vi "AlGaInPAs_v22b.vi"(2 "Debug Mode":bool, 3 "Elapsed Time(s)":dbl, 4 "State":enum16{"Edit", "Start", "Run", "End", "Idle"}(ring), 5 "Argument List In":string[](array[string])) -> (0 "Status Out":string, 1 "Argument List Out":string[](array[string]))   [LabVIEW 2011]
uses:
  high_level_proc/source_dilution.ctl
  high_level_proc/source_noDilution.ctl
panel:
  in  "Ring":u16(ring)
  out "source array":refnum<vi>[](array[refnum])
  in  "Zn bubbler":T1={"Dilution"=FALSE, "Calculated"=0, "MFC1 flow"=0.0, "MFC2 flow"=10.0, "MFC3 flow"=100.0, "Main"={"Flow"=0.0, "Prep"=FALSE, "Run"=FALSE, "Active"=FALSE, "Name"="Zn"}} caption="Al" {"Main"."Flow" format="%.2f"; "MFC1 flow" format="%.4f"; "MFC3 flow" format="%.1f"; "MFC2 flow" format="%.2f"; "Calculated" items=["Flow", "MFC1", "MFC2", "MFC3"]}
  in  "Al bubbler":T2={"Flow"=0.0, "Prep"=FALSE, "Run"=FALSE, "Active"=FALSE, "Name"="Al"} caption="Al" {"Flow" format="%.2f"}
  in  "Se bubbler":T1={"Dilution"=FALSE, "Calculated"=0, "MFC1 flow"=0.0, "MFC2 flow"=10.0, "MFC3 flow"=100.0, "Main"={"Flow"=0.0, "Prep"=FALSE, "Run"=FALSE, "Active"=FALSE, "Name"="Se"}} caption="Al" {"Main"."Flow" format="%.2f"; "MFC1 flow" format="%.4f"; "MFC3 flow" format="%.1f"; "MFC2 flow" format="%.2f"; "Calculated" items=["Flow", "MFC1", "MFC2", "MFC3"]}
  in  "P bubbler":T2={"Flow"=0.0, "Prep"=FALSE, "Run"=FALSE, "Active"=FALSE, "Name"="P liq"} caption="Al" {"Flow" format="%.2f"}
  in  "As gas":T2={"Flow"=0.0, "Prep"=FALSE, "Run"=FALSE, "Active"=FALSE, "Name"="As gas"} caption="Al" {"Flow" format="%.2f"}
  in  "P gas":T2={"Flow"=0.0, "Prep"=FALSE, "Run"=FALSE, "Active"=FALSE, "Name"="P gas"} caption="Al" {"Flow" format="%.2f"}
  in  "In bubbler":T2={"Flow"=0.0, "Prep"=FALSE, "Run"=FALSE, "Active"=FALSE, "Name"="In"} caption="Al" {"Flow" format="%.2f"}
  in  "Ga bubbler":T1={"Dilution"=FALSE, "Calculated"=0, "MFC1 flow"=0.0, "MFC2 flow"=10.0, "MFC3 flow"=100.0, "Main"={"Flow"=0.0, "Prep"=FALSE, "Run"=FALSE, "Active"=FALSE, "Name"="Ga"}} caption="Al" {"Main"."Flow" format="%.2f"; "MFC1 flow" format="%.4f"; "MFC3 flow" format="%.1f"; "MFC2 flow" format="%.2f"; "Calculated" items=["Flow", "MFC1", "MFC2", "MFC3"]}
  out "prep_done":bool
  out "run started":bool
  out "first":bool=TRUE
  out "is OK?":bool
  in  "prep_time":dbl
  in  "Cancel":bool
  in  "OK":bool
  # "s"
  # "Add pre-run time to run time in editor."
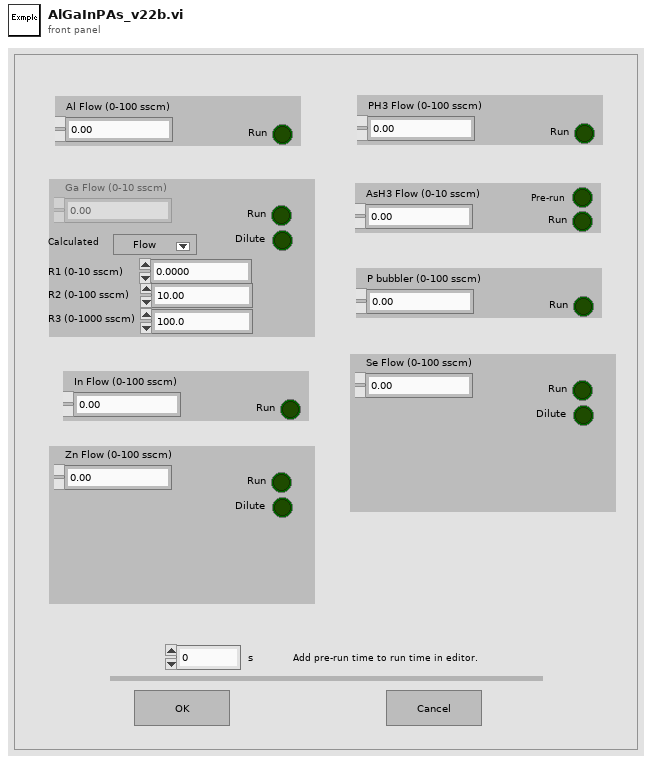
[diagram p1: front panel]
types:
  T1 = typedef "source_dilution.ctl" = cluster{"Dilution":bool, "Calculated":u16, "MFC1 flow":dbl, "MFC2 flow":dbl, "MFC3 flow":dbl, "Main":T2}
  T2 = typedef "source_noDilution.ctl" = cluster{"Flow":dbl, "Prep":bool, "Run":bool, "Active":bool, "Name":string}
  T3 = enum32{"Invalid", "Default", "Floating", "Floating/Auto-Hide", "Modal"}
  T4 = enum16{"Discrete", "Continuous", "Instantaneous", "Finite"}
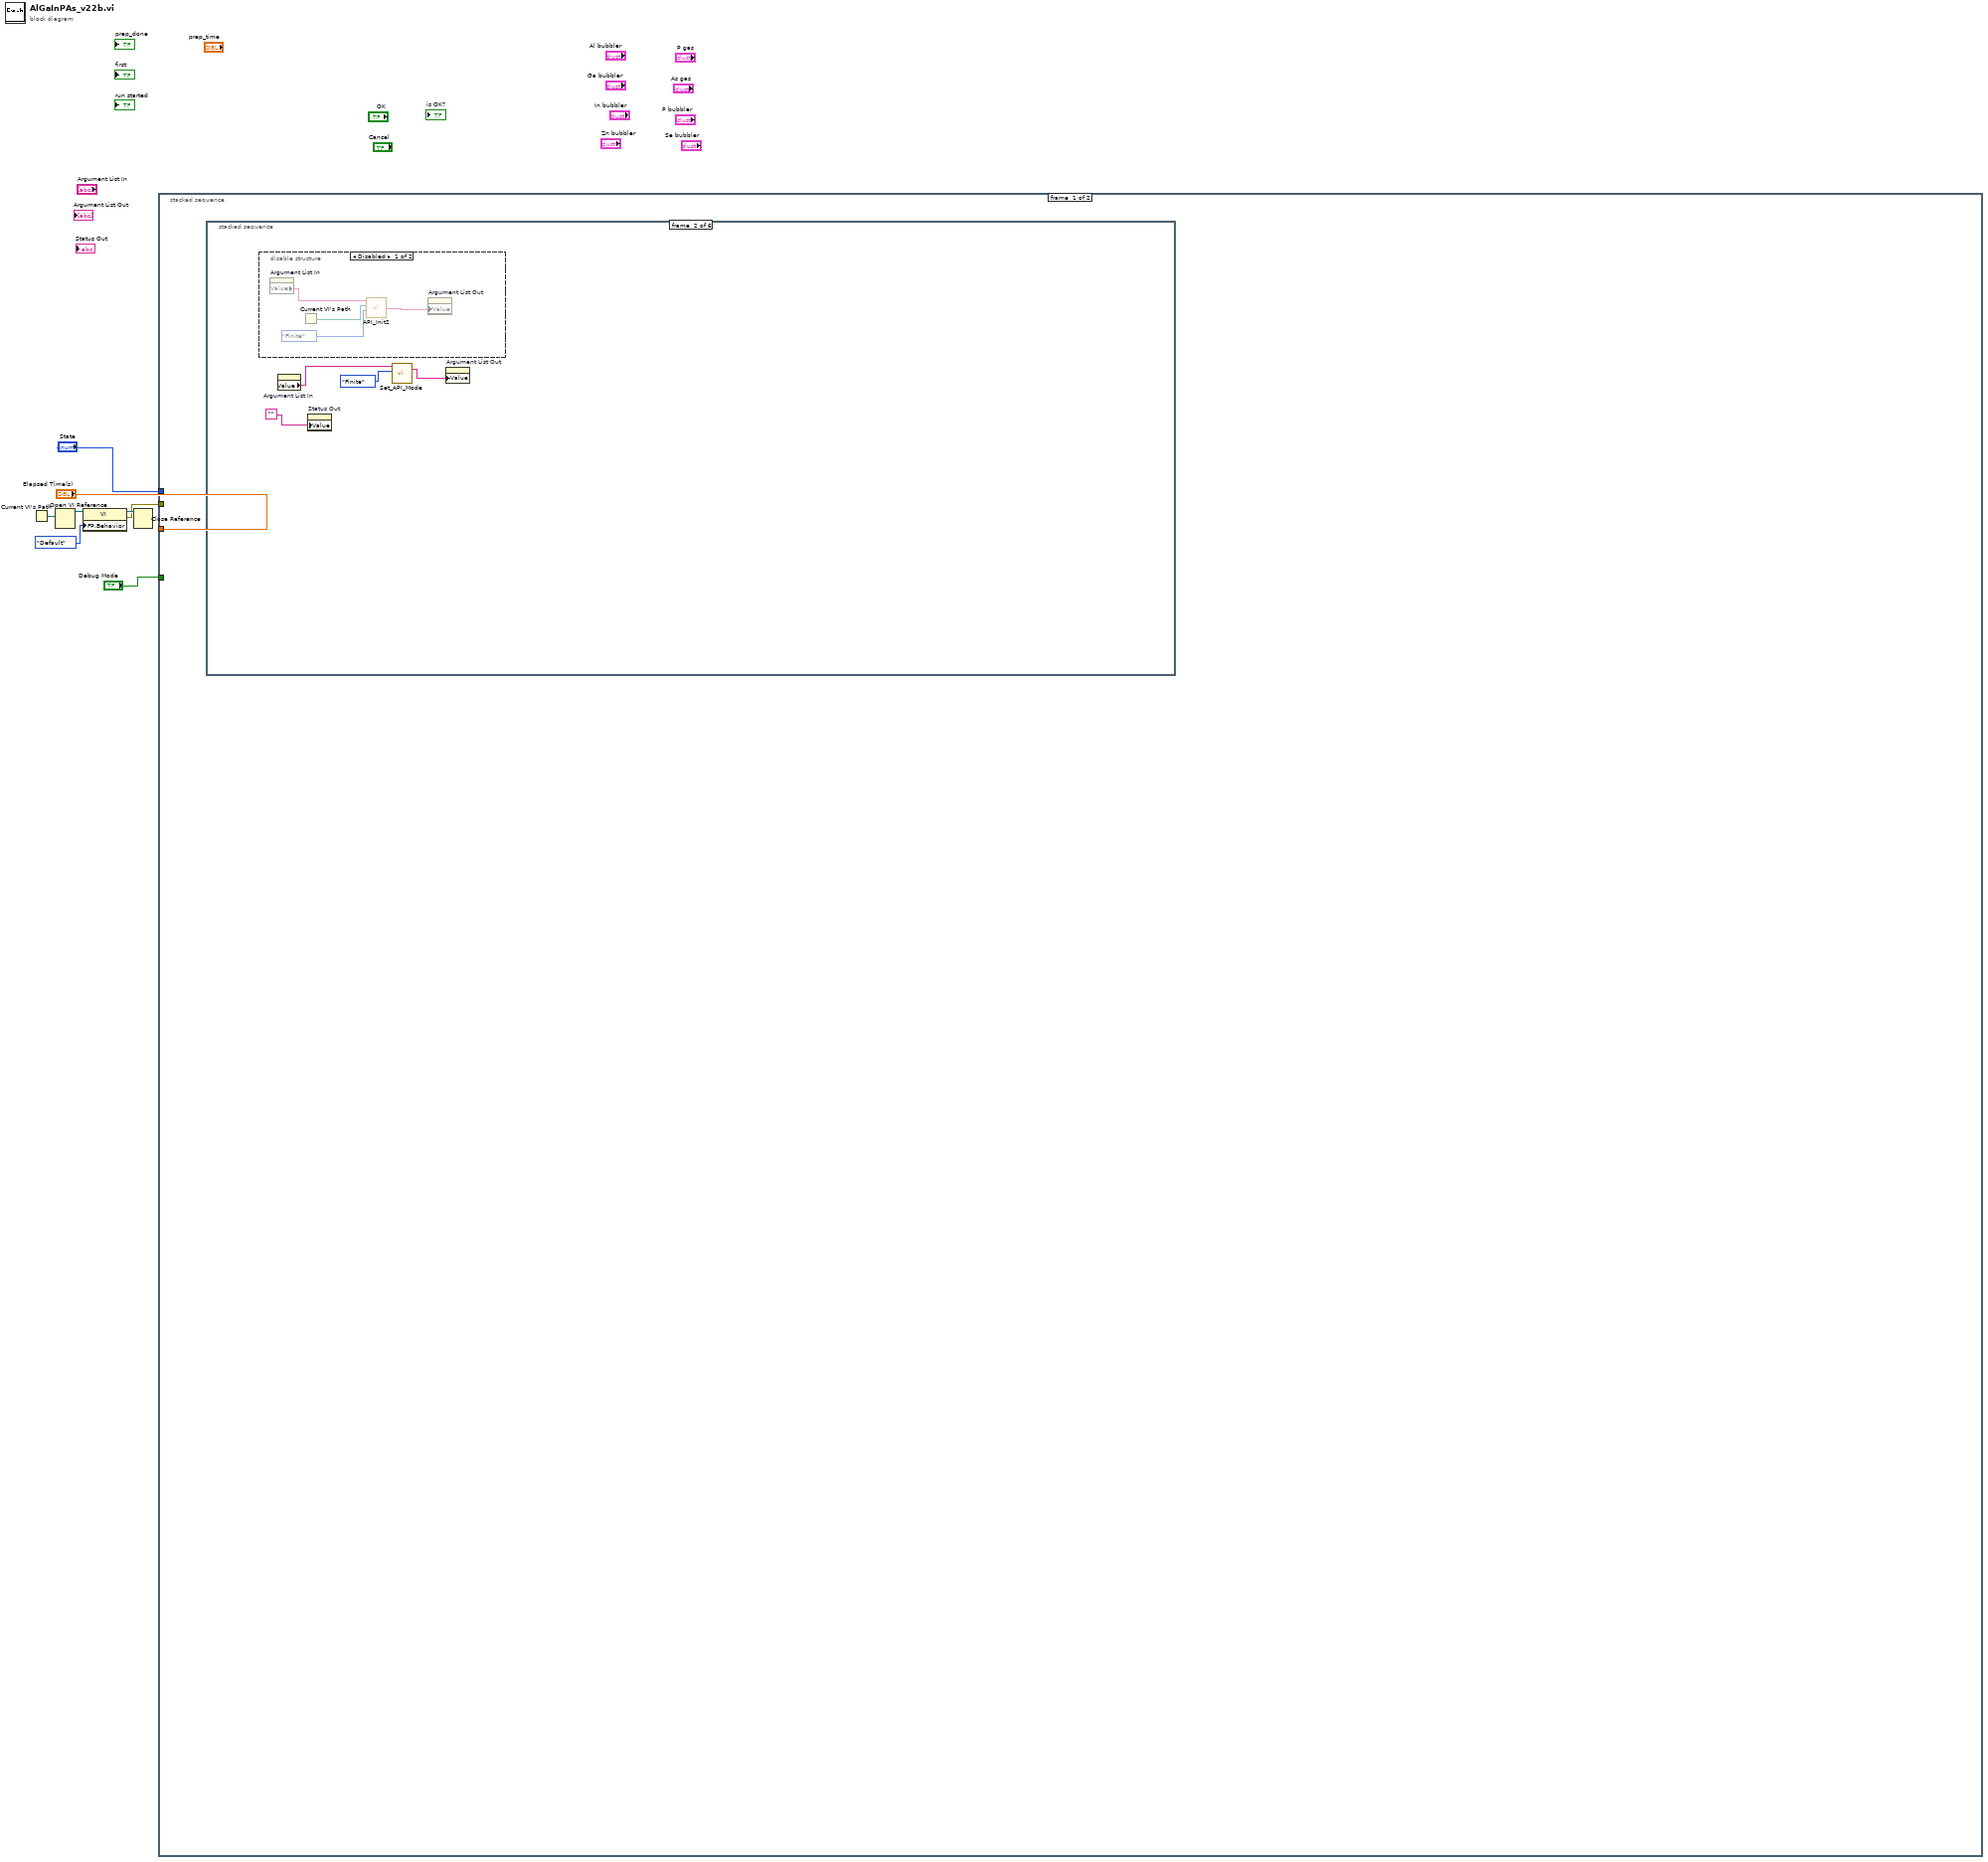
[diagram p0: block diagram]
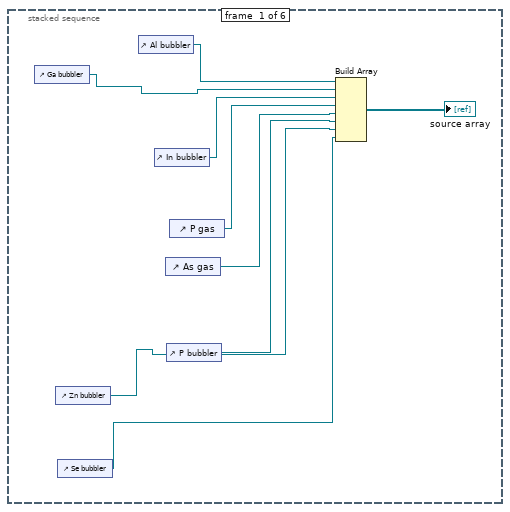
[diagram p2: hidden frame]
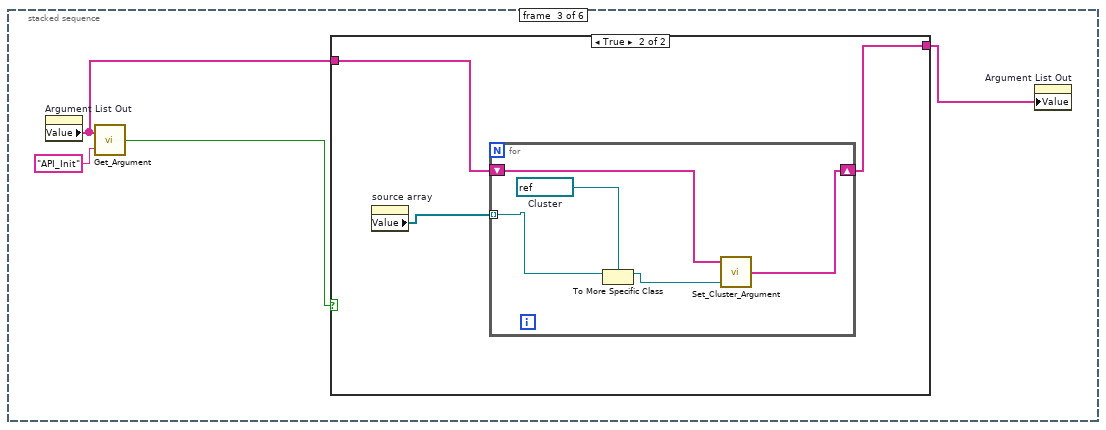
[diagram p4: hidden frame]
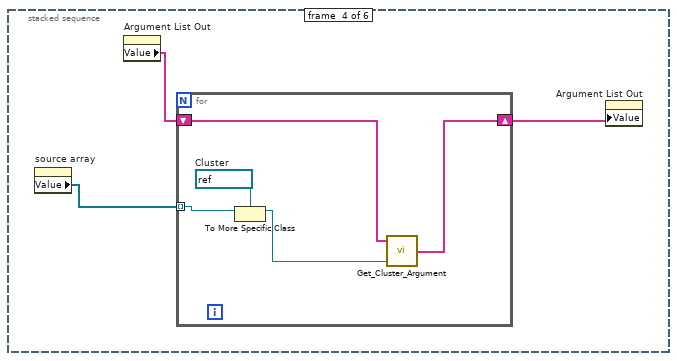
[diagram p6: hidden frame]
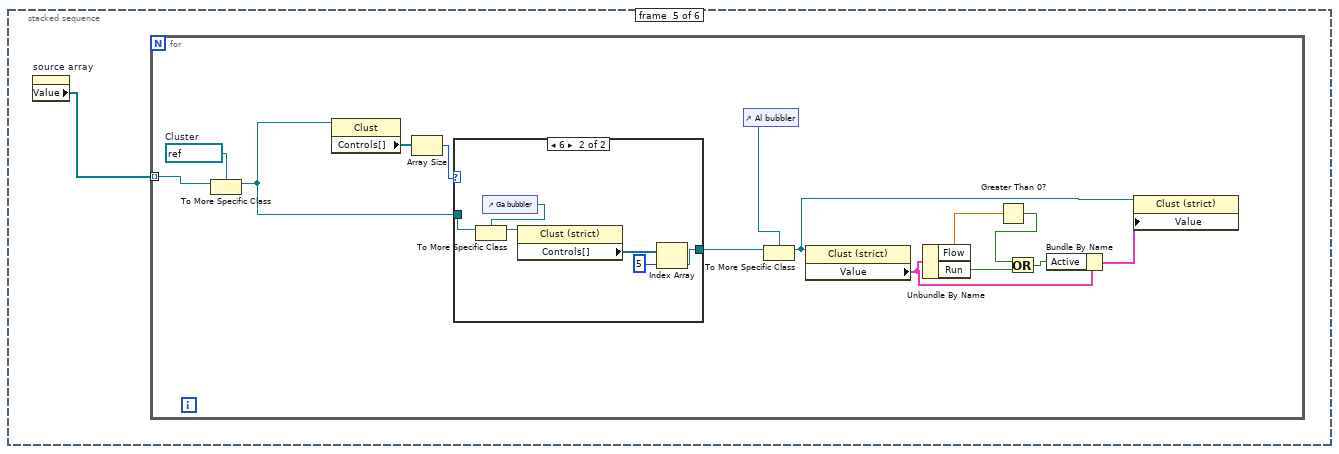
[diagram p7: hidden frame]
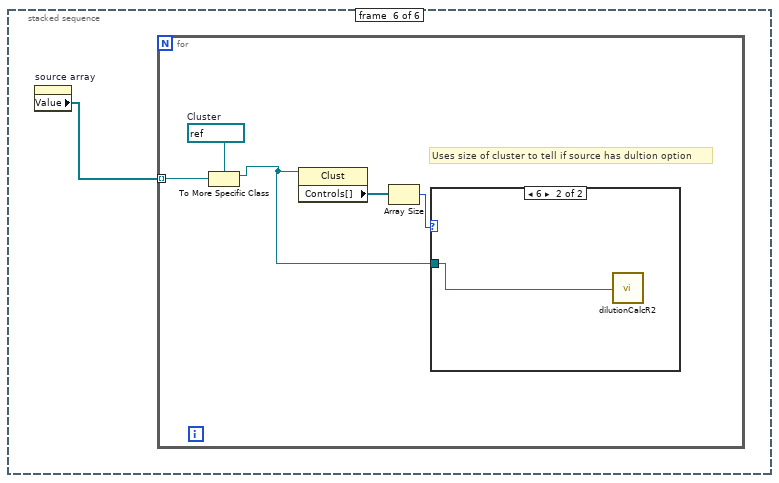
[diagram p9: hidden frame]
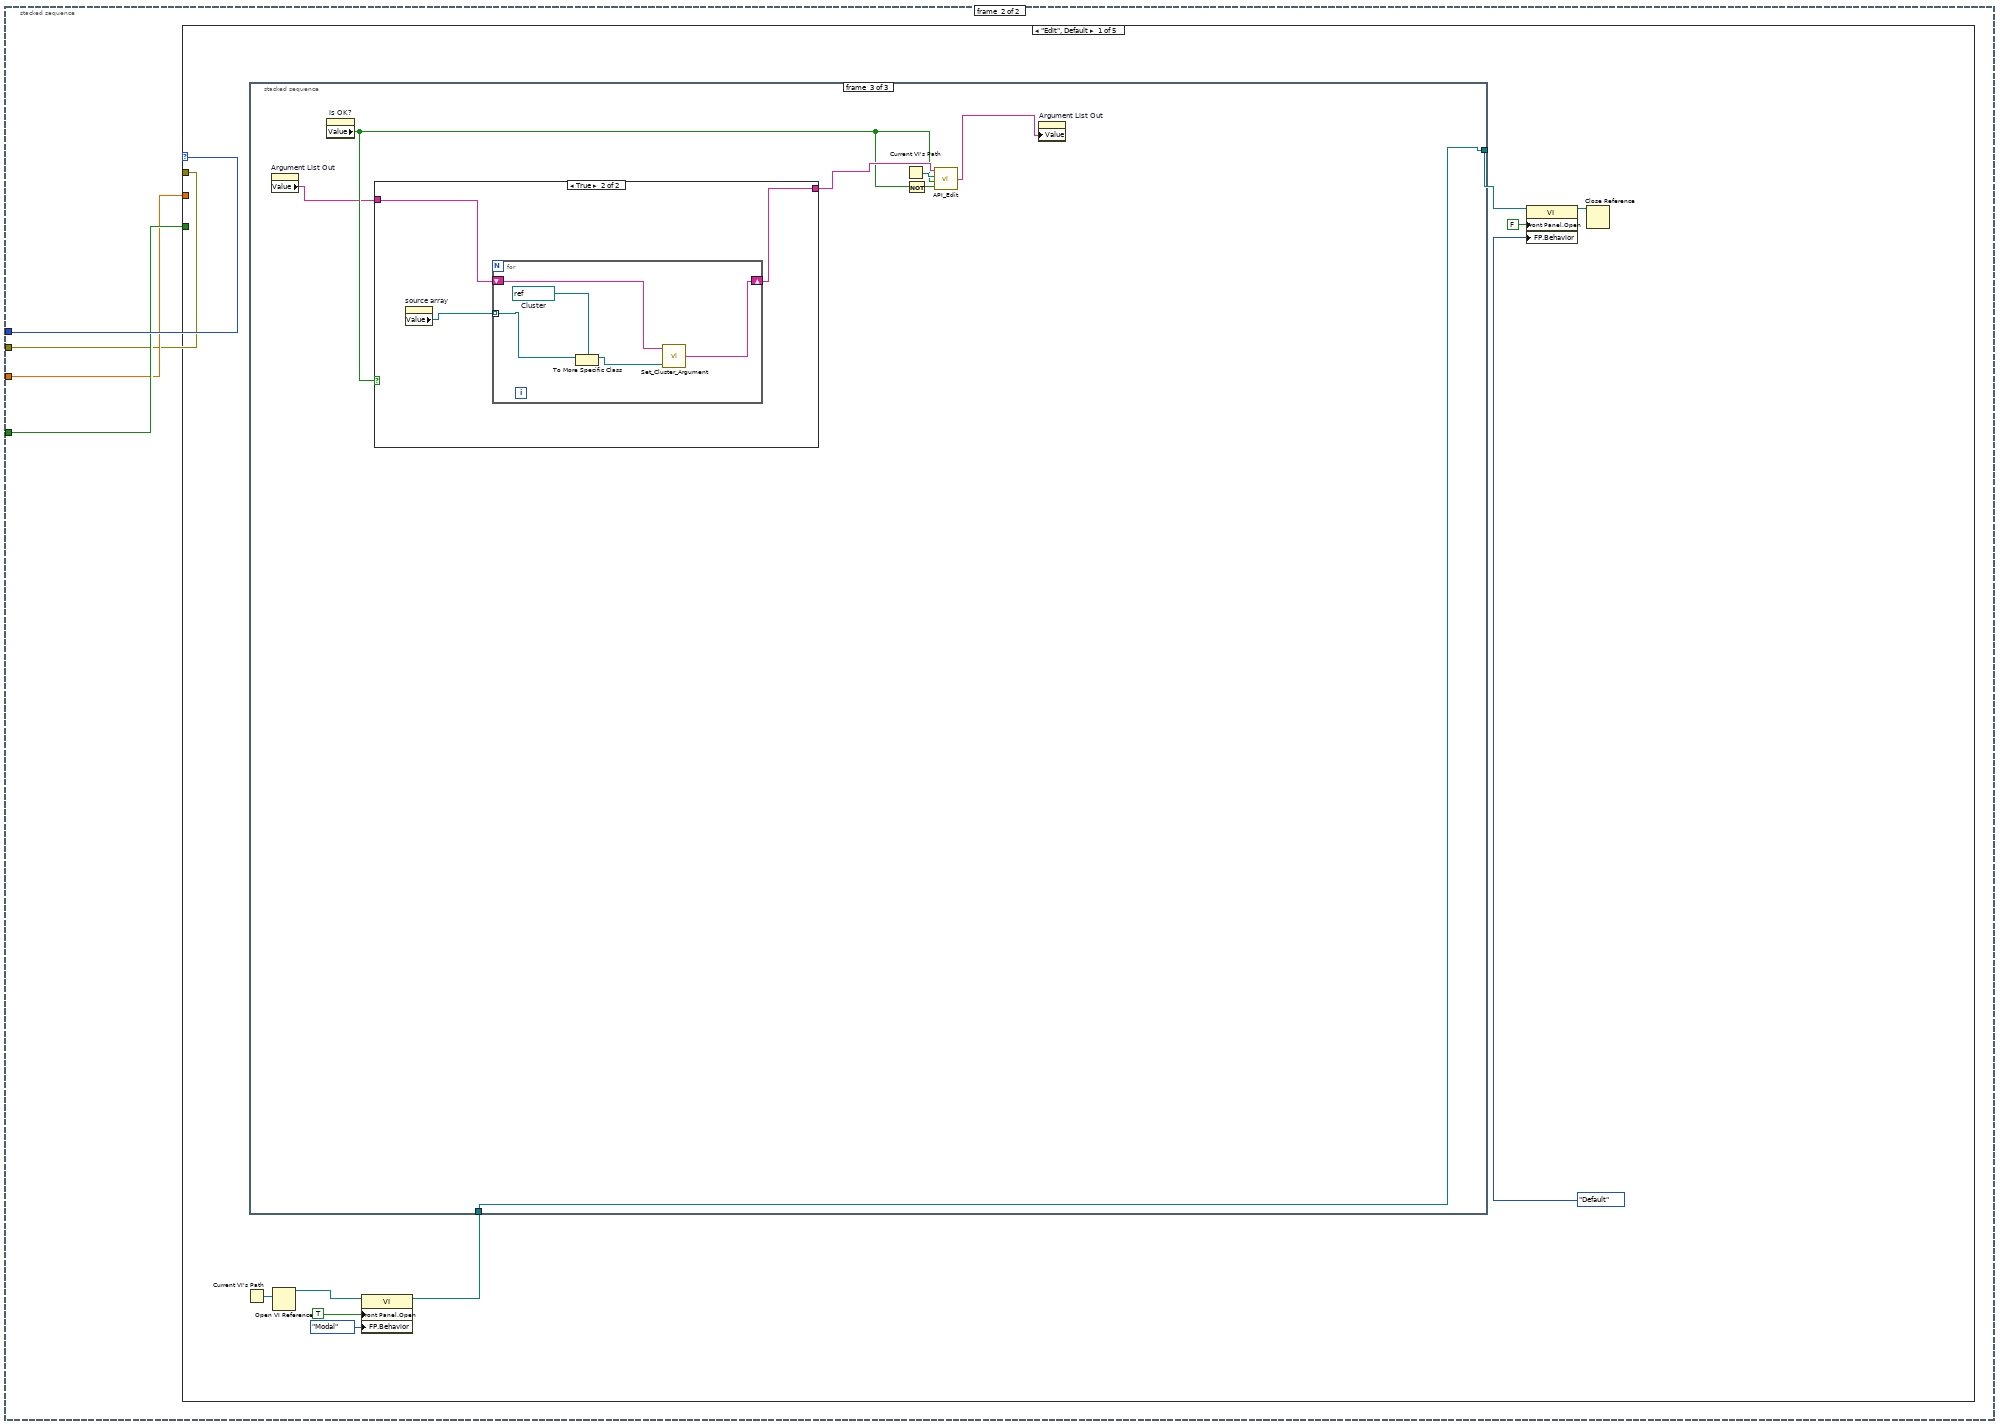
[diagram p11: hidden frame]
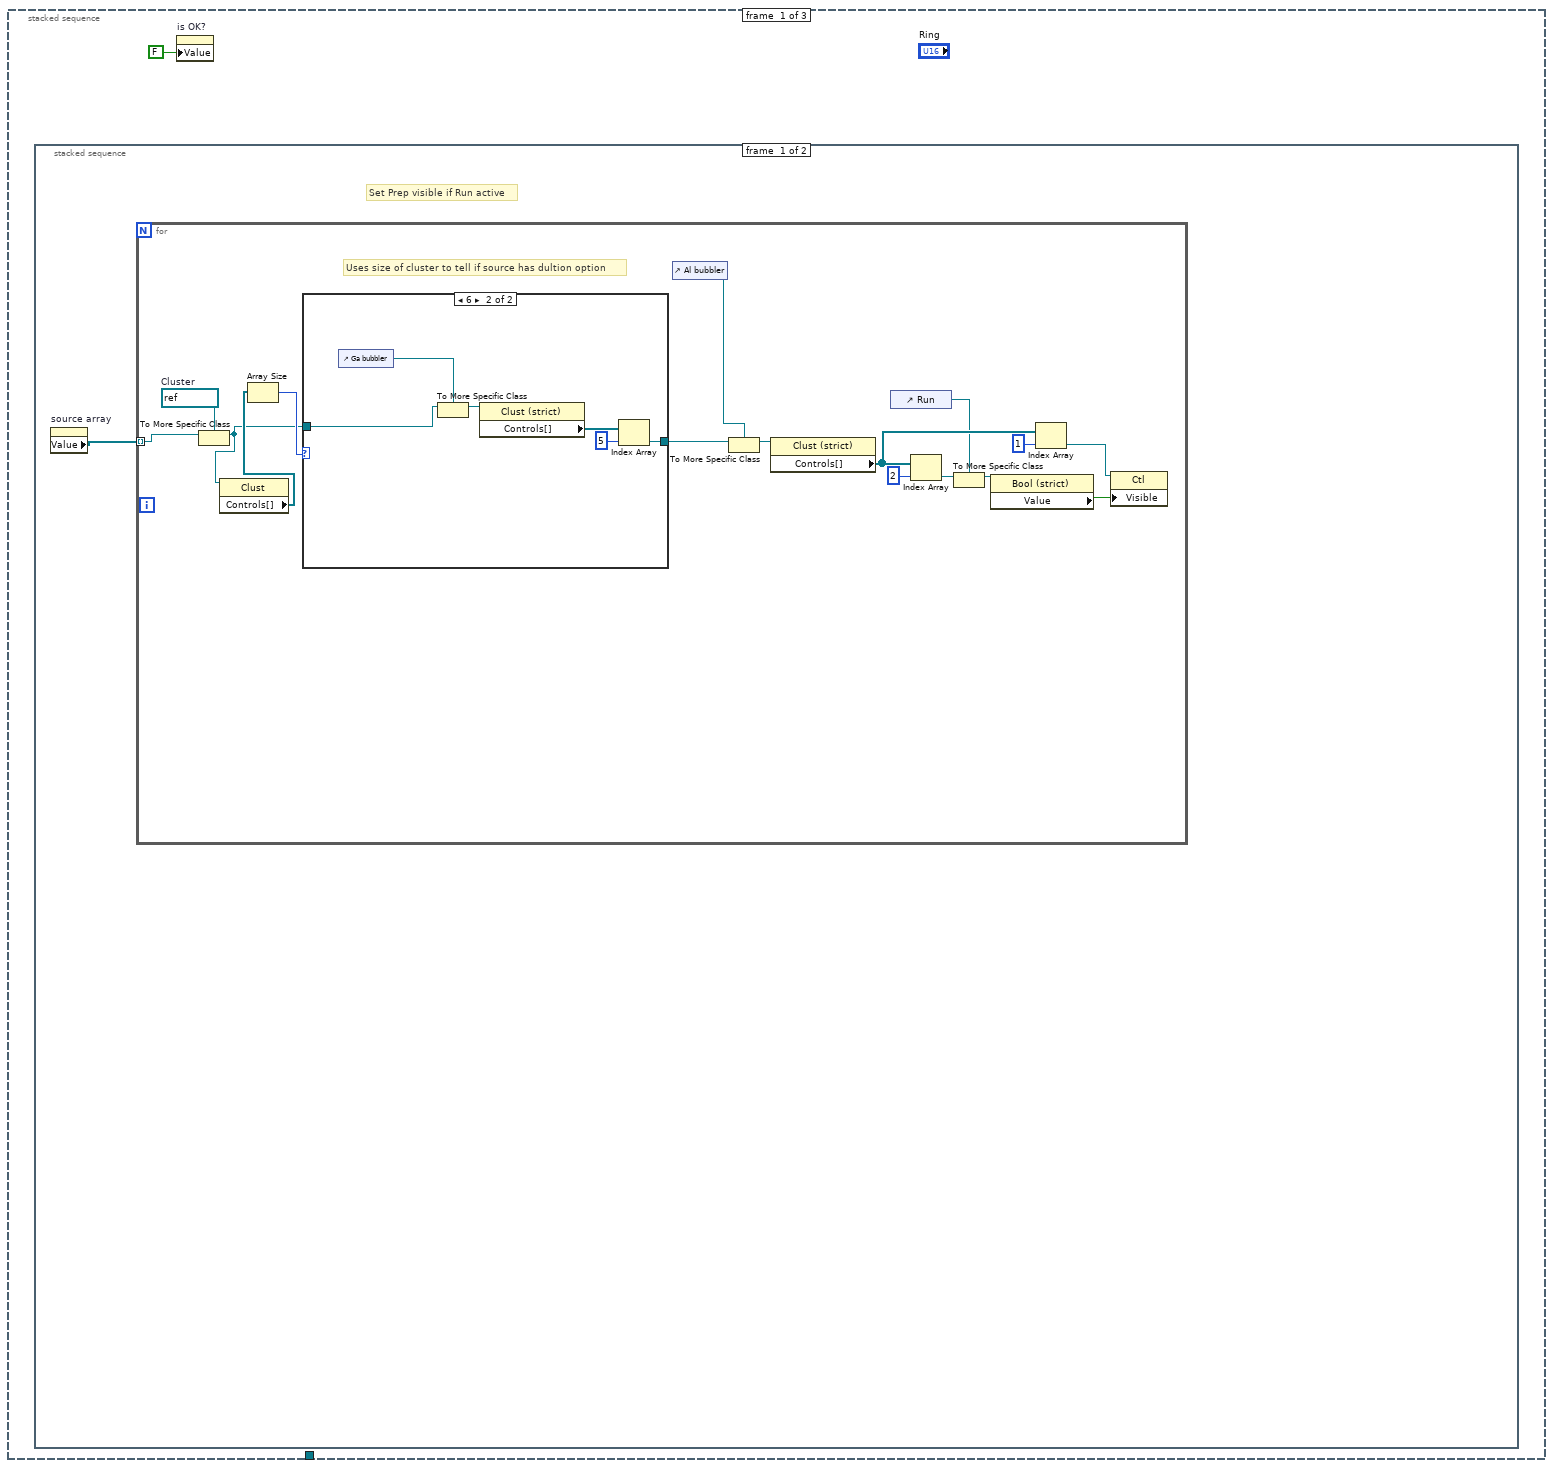
[diagram p12: hidden frame]
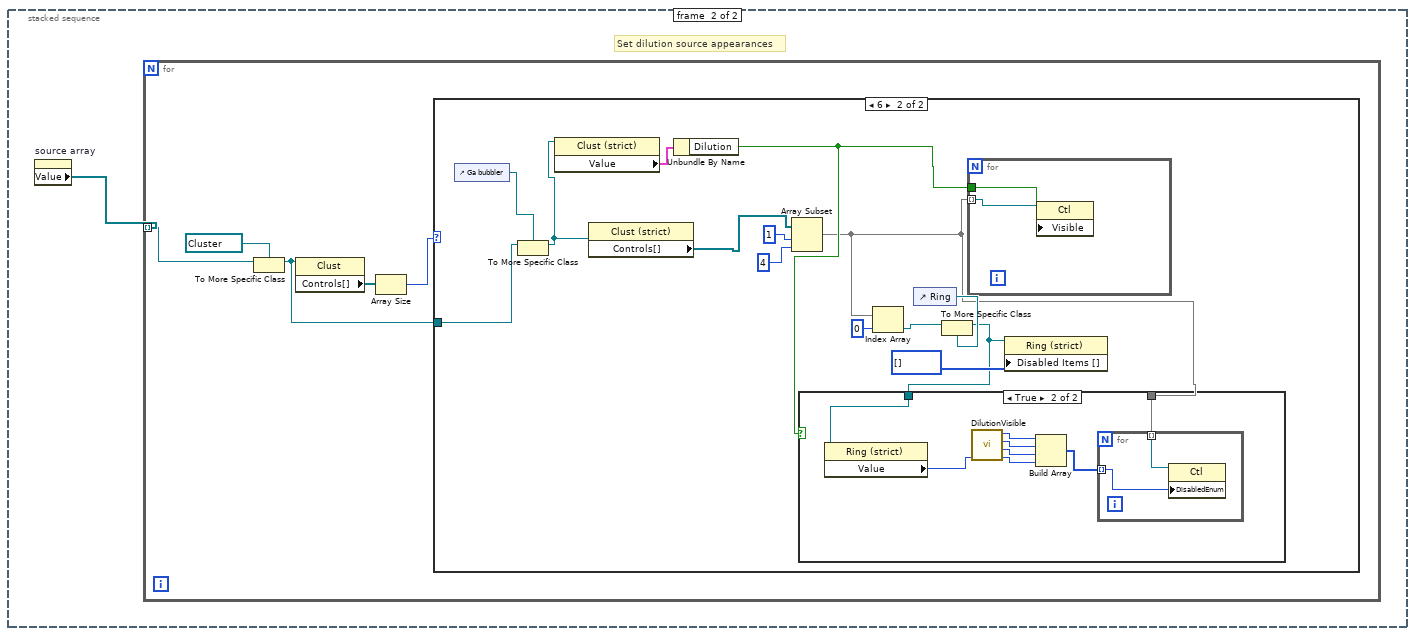
[diagram p14: hidden frame]
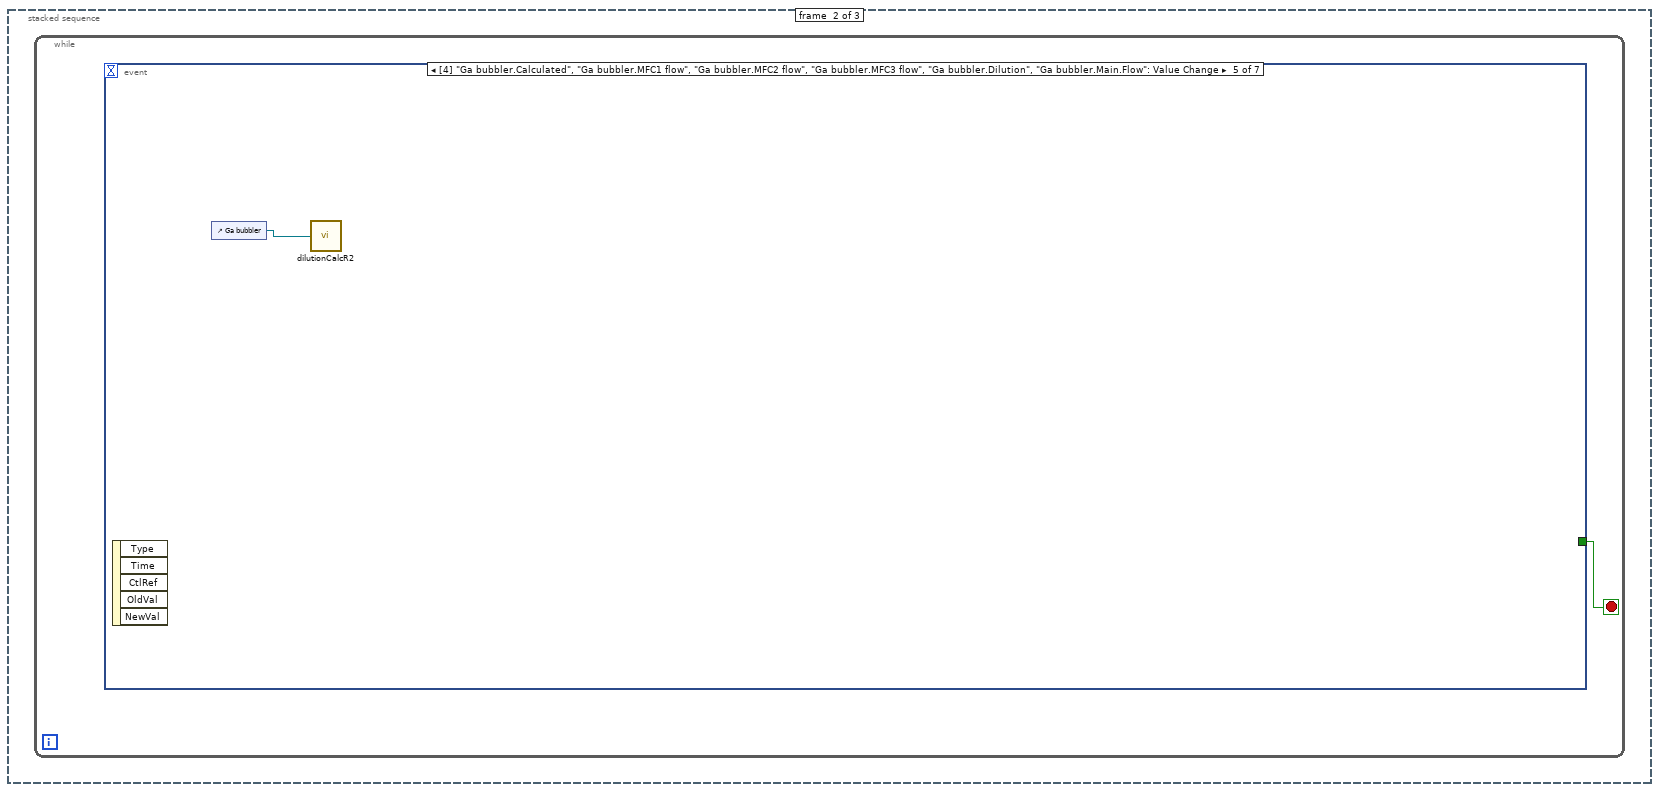
[diagram p17: hidden frame]
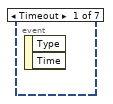
[diagram p18: hidden frame]
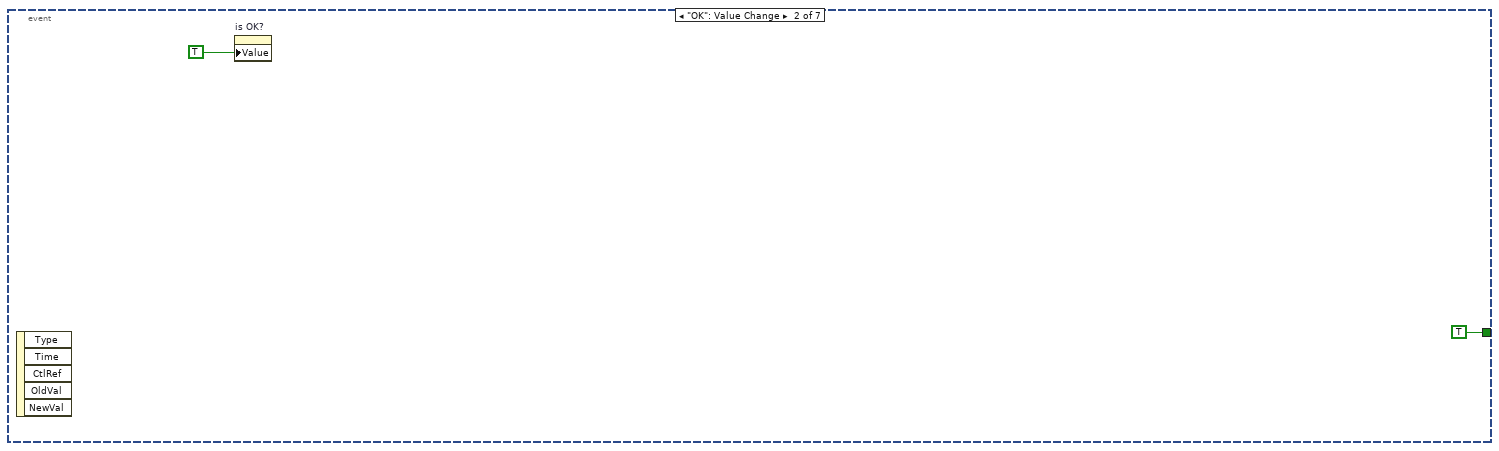
[diagram p19: hidden frame]
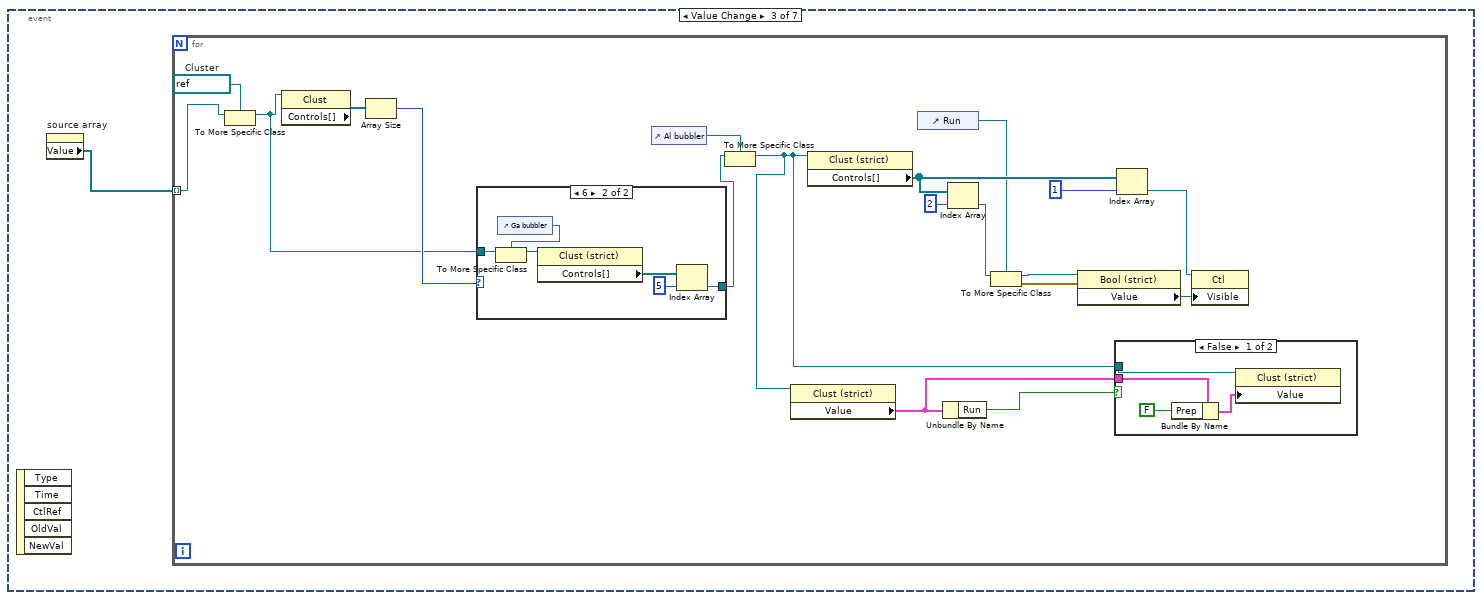
[diagram p20: hidden frame]
diagram:
  n1 = Current VI's Path() -> (path=w5:path)
  n2 = Open VI Reference(vi path=w5) -> (vi reference=w4:refnum<vi>)  [unwired: 1 in, 5 out]
  n3 = property class="VI"(reference=w4, "FP.Behavior"=T3."Default" ("Front Panel Window:Behavior")) -> (reference out=w2:refnum<vi>, error out=w1:errorcluster)  [unwired: 1 in]
  n4 = Close Reference(reference=w2) -> ()  [unwired: 1 in, 1 out]
  n5 = stacked-sequence {
    tunnel: "State" -> [_ w79]
    tunnel: "Debug Mode" -> [_ w78]
    tunnel: "Elapsed Time(s)" -> [_ w77]
    tunnel: w1 -> [_ w76]
    frame #0 {
      n6 = stacked-sequence {
        frame #0 {
          n7 = control-ref of="Ga bubbler"() -> (w12:refnum<vi>)
          n8 = control-ref of="Zn bubbler"() -> (w11:refnum<vi>)
          n9 = control-ref of="Se bubbler"() -> (w10:refnum<vi>)
          n10 = control-ref of="Al bubbler"() -> (w17:refnum<vi>)
          n11 = control-ref of="In bubbler"() -> (w16:refnum<vi>)
          n12 = control-ref of="As gas"() -> (w14:refnum<vi>)
          n13 = control-ref of="P bubbler"() -> (w13:refnum<vi>)
          n14 = control-ref of="P gas"() -> (w15:refnum<vi>)
          n15 = Build Array(w17, w12, w16, w15, w14, w13, w11, w10) -> (→"source array":refnum<vi>[])
        }
        frame #1 {
          n16 = disable-structure shown="Disabled" {
            frame Disabled {
              n17 = property on="Argument List In" class="Arr (strict)"() -> ("Value"=w25:string[])  [unwired: 2 in, 2 out]
              n18 = Current VI's Path() -> (path=w22:path)
              n19 = call "API_Init2.vi"("API Mode"=T4."Finite", "VI Path"=w22, "Argument List In"=w25) -> ("Argument List Out"=w24:string[])  [unwired: 1 in]
              n20 = property on="Argument List Out" class="Arr (strict)"("Value"=w24) -> ()  [unwired: 2 in, 2 out]
            }
            frame Enabled {
            }
          }
          n21 = property on="Argument List In" class="Arr (strict)"() -> ("Value"=w20:string[])  [unwired: 2 in, 2 out]
          n22 = property on="Status Out" class="Str"("Value"="") -> ()  [unwired: 2 in, 2 out]
          n23 = call "Set_API_Mode.vi"("API Mode"=T4."Finite", "Argument List In"=w20) -> ("Argument List Out"=w18:string[])  [unwired: 3 in]
          n24 = property on="Argument List Out" class="Arr (strict)"("Value"=w18) -> ()  [unwired: 2 in, 2 out]
        }
        frame #2 {
          n25 = property on="Argument List Out" class="Arr (strict)"() -> ("Value"=w27:string[])  [unwired: 2 in, 2 out]
          n26 = call "Get_Argument.vi"("Argument"="API_Init", "Argument List"=w27) -> ("Enabled"=w28:bool)
          n27 = case shown="True" w28 {
            tunnel: w27 -> [w30 w33]
            tunnel: [w30 w32] -> w26
            frame False {
            }
            frame True {
              n28 = property on="source array" class="Arr (strict)"() -> ("Value"=w31:refnum<vi>[])  [unwired: 2 in, 2 out]
              n29 = for {
                shift-right: [w37] -> w32
                shift-left: w33 -> [w38]
                tunnel: w31 -> [w36] mode=indexing
                w35 = refnum<vi> refnum  # Cluster
                n30 = To More Specific Class(target class=w35, reference=w36) -> (specific class reference=w34:refnum<vi>)  [unwired: 1 in, 1 out]
                n31 = call "Set_Cluster_Argument.vi"("Clust Refnum"=w34, "Argument List In"=w38) -> ("Argument List Out"=w37:string[])  [unwired: 1 in]
              }
            }
          }
          n32 = property on="Argument List Out" class="Arr (strict)"("Value"=w26) -> ()  [unwired: 2 in, 2 out]
        }
        frame #3 {
          n33 = property on="source array" class="Arr (strict)"() -> ("Value"=w39:refnum<vi>[])  [unwired: 2 in, 2 out]
          n34 = property on="Argument List Out" class="Arr (strict)"() -> ("Value"=w41:string[])  [unwired: 2 in, 2 out]
          n35 = for {
            shift-right: [w45] -> w40
            shift-left: w41 -> [w46]
            tunnel: w39 -> [w44] mode=indexing
            w42 = refnum<vi> refnum  # Cluster
            n36 = To More Specific Class(target class=w42, reference=w44) -> (specific class reference=w43:refnum<vi>)  [unwired: 1 in, 1 out]
            n37 = call "Get_Cluster_Argument.vi"("source"=w43, "Argument List In"=w46) -> ("Argument List Out"=w45:string[])  [unwired: 1 in]
          }
          n38 = property on="Argument List Out" class="Arr (strict)"("Value"=w40) -> ()  [unwired: 2 in, 2 out]
        }
        frame #4 {
          n39 = property on="source array" class="Arr (strict)"() -> ("Value"=w47:refnum<vi>[])  [unwired: 2 in, 2 out]
          n40 = for {
            tunnel: w47 -> [w50] mode=indexing
            w48 = refnum<vi> refnum  # Cluster
            n41 = To More Specific Class(target class=w48, reference=w50) -> (specific class reference=w49:refnum<vi>)  [unwired: 1 in, 1 out]
            n42 = property class="Clust"(reference=w49) -> ("Controls[]"=w52:refnum<vi>[])  [unwired: 1 in, 2 out]
            n43 = Array Size(array=w52) -> (size(s)=w53:i32)
            n44 = case shown="6" w53 {
              tunnel: [w62 w64] -> w51
              tunnel: w49 -> [w62 w67]
              frame Default {
              }
              frame 6 {
                n45 = control-ref of="Ga bubbler"() -> (w63:refnum<vi>)
                n46 = To More Specific Class(target class=w63, reference=w67) -> (specific class reference=w66:refnum<vi>)  [unwired: 1 in, 1 out]
                n47 = property class="Clust (strict)"(reference=w66) -> ("Controls[]"=w65:refnum<vi>[])  [unwired: 1 in, 2 out]
                n48 = Index Array(array=w65, index=5) -> (element=w64:refnum<vi>)
              }
            }
            n49 = control-ref of="Al bubbler"() -> (w55:refnum<vi>)
            n50 = To More Specific Class(target class=w55, reference=w51) -> (specific class reference=w54:refnum<vi>)  [unwired: 1 in, 1 out]
            n51 = property class="Clust (strict)"(reference=w54) -> ("Value"=w58:T2)  [unwired: 1 in, 2 out]
            n52 = Unbundle By Name(w58) -> ("Flow"=w61:dbl, "Run"=w59:bool)
            n53 = Greater Than 0?(x=w61) -> (x > 0?=w60:bool)
            n54 = Or(x=w60, y=w59) -> (x .or. y?=w56:bool)
            n55 = Bundle By Name(cluster=w58, "Active"=w56) -> (w57:T2)
            n56 = property class="Clust (strict)"(reference=w54, "Value"=w57) -> ()  [unwired: 1 in, 2 out]
          }
        }
        frame #5 {
          n57 = property on="source array" class="Arr (strict)"() -> ("Value"=w69:refnum<vi>[])  [unwired: 2 in, 2 out]
          n58 = for {
            tunnel: w69 -> [w73] mode=indexing
            w71 = refnum<vi> refnum  # Cluster
            # "Uses size of cluster to tell if source has dultion option"
            n59 = To More Specific Class(target class=w71, reference=w73) -> (specific class reference=w72:refnum<vi>)  [unwired: 1 in, 1 out]
            n60 = property class="Clust"(reference=w72) -> ("Controls[]"=w70:refnum<vi>[])  [unwired: 1 in, 2 out]
            n61 = Array Size(array=w70) -> (size(s)=w74:i32)
            n62 = case shown="6" w74 {
              tunnel: w72 -> [_ w75]
              frame Default {
              }
              frame 6 {
                n63 = call "dilutionCalcR2.vi"("Clust Refnum"=w75) -> ()
              }
            }
          }
        }
      }
    }
    frame #1 {
      n64 = case shown="\"Edit\", Default" w79 {
        tunnel: w78 -> [_ w203 w219 _ _]
        tunnel: w77 -> [_ _ w220 _ _]
        tunnel: w76 -> [_ _ _ _ _]
        frame "Edit", Default {
          n65 = Current VI's Path() -> (path=w84:path)
          n66 = Open VI Reference(vi path=w84) -> (vi reference=w83:refnum<vi>)  [unwired: 1 in, 5 out]
          n67 = property class="VI"(reference=w83, "Front Panel.Open"=TRUE ("Front Panel Window:Open"), "FP.Behavior"=T3."Modal" ("Front Panel Window:Behavior")) -> (reference out=w81:refnum<vi>)  [unwired: 1 in, 1 out]
          n68 = stacked-sequence {
            tunnel: [_ _ w186] -> w86
            tunnel: w81 -> [_ _ w186]
            frame #0 {
              n69 = stacked-sequence {
                frame #0 {
                  # "Set Prep visible if Run active"
                  n70 = property on="source array" class="Arr (strict)"() -> ("Value"=w90:refnum<vi>[])  [unwired: 2 in, 2 out]
                  n71 = for {
                    tunnel: w90 -> [w95] mode=indexing
                    w94 = refnum<vi> refnum  # Cluster
                    # "Uses size of cluster to tell if source has dultion option"
                    n72 = To More Specific Class(target class=w94, reference=w95) -> (specific class reference=w91:refnum<vi>)  [unwired: 1 in, 1 out]
                    n73 = property class="Clust"(reference=w91) -> ("Controls[]"=w93:refnum<vi>[])  [unwired: 1 in, 2 out]
                    n74 = Array Size(array=w93) -> (size(s)=w92:i32)
                    n75 = case shown="6" w92 {
                      tunnel: w91 -> [w107 w110]
                      tunnel: [w107 w111] -> w97
                      frame Default {
                      }
                      frame 6 {
                        n76 = control-ref of="Ga bubbler"() -> (w108:refnum<vi>)
                        n77 = To More Specific Class(target class=w108, reference=w110) -> (specific class reference=w109:refnum<vi>)  [unwired: 1 in, 1 out]
                        n78 = property class="Clust (strict)"(reference=w109) -> ("Controls[]"=w113:refnum<vi>[])  [unwired: 1 in, 2 out]
                        n79 = Index Array(array=w113, index=5) -> (element=w111:refnum<vi>)
                      }
                    }
                    n80 = control-ref of="Al bubbler"() -> (w98:refnum<vi>)
                    n81 = To More Specific Class(target class=w98, reference=w97) -> (specific class reference=w104:refnum<vi>)  [unwired: 1 in, 1 out]
                    n82 = property class="Clust (strict)"(reference=w104) -> ("Controls[]"=w103:refnum<vi>[])  [unwired: 1 in, 2 out]
                    n83 = control-ref of="Run"() -> (w96:refnum<vi>)
                    n84 = Index Array(array=w103, index=2) -> (element=w101:refnum<vi>)
                    n85 = To More Specific Class(target class=w96, reference=w101) -> (specific class reference=w100:refnum<vi>)  [unwired: 1 in, 1 out]
                    n86 = property class="Bool (strict)"(reference=w100) -> ("Value"=w99:bool)  [unwired: 1 in, 2 out]
                    n87 = Index Array(array=w103, index=1) -> (element=w105:refnum<vi>)
                    n88 = property class="Ctl"(reference=w105, "Visible"=w99) -> ()  [unwired: 1 in, 2 out]
                  }
                }
                frame #1 {
                  # "Set dilution source appearances"
                  n89 = property on="source array" class="Arr (strict)"() -> ("Value"=w114:refnum<vi>[])  [unwired: 2 in, 2 out]
                  n90 = for {
                    tunnel: w114 -> [w119] mode=indexing
                    n91 = To More Specific Class(target class=refnum<vi> refnum, reference=w119) -> (specific class reference=w115:refnum<vi>)  [unwired: 1 in, 1 out]
                    n92 = property class="Clust"(reference=w115) -> ("Controls[]"=w117:refnum<vi>[])  [unwired: 1 in, 2 out]
                    n93 = Array Size(array=w117) -> (size(s)=w116:i32)
                    n94 = case shown="6" w116 {
                      tunnel: w115 -> [_ w133]
                      frame Default {
                      }
                      frame 6 {
                        n95 = control-ref of="Ga bubbler"() -> (w132:refnum<vi>)
                        n96 = To More Specific Class(target class=w132, reference=w133) -> (specific class reference=w130:refnum<vi>)  [unwired: 1 in, 1 out]
                        n97 = property class="Clust (strict)"(reference=w130) -> ("Value"=w131:T1)  [unwired: 1 in, 2 out]
                        n98 = property class="Clust (strict)"(reference=w130) -> ("Controls[]"=w129:refnum<vi>[])  [unwired: 1 in, 2 out]
                        n99 = Unbundle By Name(w131) -> ("Dilution"=w123:bool)
                        n100 = Array Subset(array=w129, index=1, length=4) -> (w120:refnum<vi>[])
                        n101 = Index Array(array=w120, index=0) -> (element=w122:refnum<vi>)
                        n102 = control-ref of="Ring"() -> (w125:refnum<vi>)
                        n103 = To More Specific Class(target class=w125, reference=w122) -> (specific class reference=w121:refnum<vi>)  [unwired: 1 in, 1 out]
                        n104 = case shown="True" w123 {
                          tunnel: w121 -> [_ w141]
                          tunnel: w120 -> [_ w134]
                          frame False {
                          }
                          frame True {
                            n105 = property class="Ring (strict)"(reference=w141) -> ("Value"=w140:u16)  [unwired: 1 in, 2 out]
                            n106 = call "DilutionVisible.vi"("calculated"=w140) -> ("MFC3"=w136:u16, "MFC2"=w137:u16, "MFC1"=w138:u16, "flow"=w139:u16)  [unwired: 3 in]
                            n107 = Build Array(w139, w138, w137, w136) -> (w135:u16[])
                            n108 = for {
                              tunnel: w135 -> [w142] mode=indexing
                              tunnel: w134 -> [w143] mode=indexing
                              n109 = property class="Ctl"(reference=w143, "DisabledEnum"=w142) -> ()  [unwired: 1 in, 2 out]
                            }
                          }
                        }
                        n110 = for {
                          tunnel: w120 -> [w145] mode=indexing
                          tunnel: w123 -> [w144]
                          n111 = property class="Ctl"(reference=w145, "Visible"=w144) -> ()  [unwired: 1 in, 2 out]
                        }
                        n112 = property class="Ring (strict)"(reference=w121, "Disabled Items []"=i32[] []) -> ()  [unwired: 1 in, 2 out]
                      }
                    }
                  }
                }
              }
              n113 = property on="is OK?" class="Bool (strict)"("Value"=FALSE ("is OK?")) -> ()  [unwired: 2 in, 2 out]
            }
            frame #1 {
              n114 = while {
                stop <- w146 stop-if-true
                n115 = event shown="[4] \"Ga bubbler.Calculated\", \"Ga bubbler.MFC1 flow\", \"Ga bubbler.MFC2 flow\", \"Ga bubbler.MFC3 flow\", \"Ga bubbler.Dilution\", \"Ga bubbler.Main.Flow\": Value Change" {
                  selector: _ -> [_ _ _ _ _ _ _]
                  dyn-events: _ -> [_ _ _ _ _ _ _]
                  timeout: _ -> [_ _ _ _ _ _ _]
                  tunnel: [_ TRUE _ TRUE _ _ _] -> w146
                  event Timeout {
                    n116 = event-data() -> ()  [unwired: 1 in, 2 out]
                  }
                  event "OK": Value Change {
                    n117 = event-data() -> ()  [unwired: 1 in, 5 out]
                    n118 = property on="is OK?" class="Bool (strict)"("Value"=TRUE ("is OK?")) -> ()  [unwired: 2 in, 2 out]
                  }
                  event Value Change {
                    n119 = event-data() -> ()  [unwired: 1 in, 5 out]
                    n120 = property on="source array" class="Arr (strict)"() -> ("Value"=w149:refnum<vi>[])  [unwired: 2 in, 2 out]
                    n121 = for {
                      tunnel: w149 -> [w152] mode=indexing
                      w150 = refnum<vi> refnum  # Cluster
                      n122 = To More Specific Class(target class=w150, reference=w152) -> (specific class reference=w151:refnum<vi>)  [unwired: 1 in, 1 out]
                      n123 = property class="Clust"(reference=w151) -> ("Controls[]"=w154:refnum<vi>[])  [unwired: 1 in, 2 out]
                      n124 = Array Size(array=w154) -> (size(s)=w153:i32)
                      n125 = case shown="6" w153 {
                        tunnel: w151 -> [w169 w172]
                        tunnel: [w169 w173] -> w156
                        frame Default {
                        }
                        frame 6 {
                          n126 = control-ref of="Ga bubbler"() -> (w170:refnum<vi>)
                          n127 = To More Specific Class(target class=w170, reference=w172) -> (specific class reference=w171:refnum<vi>)  [unwired: 1 in, 1 out]
                          n128 = property class="Clust (strict)"(reference=w171) -> ("Controls[]"=w175:refnum<vi>[])  [unwired: 1 in, 2 out]
                          n129 = Index Array(array=w175, index=5) -> (element=w173:refnum<vi>)
                        }
                      }
                      n130 = control-ref of="Al bubbler"() -> (w160:refnum<vi>)
                      n131 = To More Specific Class(target class=w160, reference=w156) -> (specific class reference=w157:refnum<vi>)  [unwired: 1 in, 1 out]
                      n132 = property class="Clust (strict)"(reference=w157) -> ("Value"=w159:T2)  [unwired: 1 in, 2 out]
                      n133 = property class="Clust (strict)"(reference=w157) -> ("Controls[]"=w166:refnum<vi>[])  [unwired: 1 in, 2 out]
                      n134 = control-ref of="Run"() -> (w155:refnum<vi>)
                      n135 = Unbundle By Name(w159) -> ("Run"=w158:bool)
                      n136 = Index Array(array=w166, index=2) -> (element=w164:refnum<vi>)
                      n137 = To More Specific Class(target class=w155, reference=w164) -> (specific class reference=w163:refnum<vi>, error out=w162:errorcluster)  [unwired: 1 in]
                      n138 = property class="Bool (strict)"(reference=w163, error in=w162) -> ("Value"=w161:bool)  [unwired: 2 out]
                      n139 = case shown="False" w158 {
                        tunnel: w159 -> [w179 _]
                        tunnel: w157 -> [w176 _]
                        frame False {
                          n140 = Bundle By Name(cluster=w179, "Prep"=FALSE) -> (w177:T2)
                          n141 = property class="Clust (strict)"(reference=w176, "Value"=w177) -> ()  [unwired: 1 in, 2 out]
                        }
                        frame True {
                        }
                      }
                      n142 = Index Array(array=w166, index=1) -> (element=w167:refnum<vi>)
                      n143 = property class="Ctl"(reference=w167, "Visible"=w161) -> ()  [unwired: 1 in, 2 out]
                    }
                  }
                  event "Cancel": Value Change {
                    n144 = event-data() -> ()  [unwired: 1 in, 5 out]
                  }
                  event Value Change {
                    n145 = event-data() -> ()  [unwired: 1 in, 5 out]
                    n146 = control-ref of="Ga bubbler"() -> (w181:refnum<vi>)
                    n147 = call "dilutionCalcR2.vi"("Clust Refnum"=w181) -> ()
                  }
                  event Value Change {
                    n148 = event-data() -> ()  [unwired: 1 in, 5 out]
                    n149 = control-ref of="Se bubbler"() -> (w182:refnum<vi>)
                    n150 = call "dilutionCalcR2.vi"("Clust Refnum"=w182) -> ()
                  }
                  event Value Change {
                    n151 = event-data() -> ()  [unwired: 1 in, 5 out]
                    n152 = control-ref of="Zn bubbler"() -> (w183:refnum<vi>)
                    n153 = call "dilutionCalcR2.vi"("Clust Refnum"=w183) -> ()
                  }
                }
              }
            }
            frame #2 {
              n154 = property on="Argument List Out" class="Arr (strict)"() -> ("Value"=w185:string[])  [unwired: 2 in, 2 out]
              n155 = property on="is OK?" class="Bool (strict)"() -> ("Value"=w187:bool)  [unwired: 2 in, 2 out]
              n156 = case shown="True" w187 {
                tunnel: w185 -> [w191 w194]
                tunnel: [w191 w193] -> w188
                frame False {
                }
                frame True {
                  n157 = property on="source array" class="Arr (strict)"() -> ("Value"=w192:refnum<vi>[])  [unwired: 2 in, 2 out]
                  n158 = for {
                    shift-right: [w198] -> w193
                    shift-left: w194 -> [w199]
                    tunnel: w192 -> [w197] mode=indexing
                    w196 = refnum<vi> refnum  # Cluster
                    n159 = To More Specific Class(target class=w196, reference=w197) -> (specific class reference=w195:refnum<vi>)  [unwired: 1 in, 1 out]
                    n160 = call "Set_Cluster_Argument.vi"("Clust Refnum"=w195, "Argument List In"=w199) -> ("Argument List Out"=w198:string[])  [unwired: 1 in]
                  }
                }
              }
              n161 = Current VI's Path() -> (path=w189:path)
              n162 = Not(x=w187) -> (.not. x?=w190:bool)
              n163 = call "API_Edit.vi"("Cancel"=w190, "OK"=w187, "VI Path"=w189, "Argument List In"=w188) -> ("Argument List Out"=w184:string[])
              n164 = property on="Argument List Out" class="Arr (strict)"("Value"=w184) -> ()  [unwired: 2 in, 2 out]
            }
          }
          n165 = property class="VI"(reference=w86, "Front Panel.Open"=FALSE ("Front Panel Window:Open"), "FP.Behavior"=T3."Default" ("Front Panel Window:Behavior")) -> (reference out=w87:refnum<vi>)  [unwired: 1 in, 1 out]
          n166 = Close Reference(reference=w87) -> ()  [unwired: 1 in, 1 out]
        }
        frame "Start" {
          n167 = property on="prep_time" class="DigNum (strict)"() -> ("Value"=w206:dbl)  [unwired: 2 in, 2 out]
          n168 = Greater Than 0?(x=w206) -> (x > 0?=w205:bool)
          n169 = Not(x=w203) -> (.not. x?=w202:bool)
          n170 = property on="Argument List Out" class="Arr (strict)"() -> ("Value"=w201:string[])  [unwired: 2 in, 2 out]
          n171 = And(x=w202, y=w205) -> (x .and. y?=w204:bool)
          n172 = call "Set_Argument.vi"("Enable"=FALSE, "Argument"="run_started", "Argument List In"=w201) -> ("Argument List Out"=w200:string[])
          n173 = case shown="True" w204 {
            frame False {
            }
            frame True {
              n174 = property on="Ga bubbler" class="Clust (strict)"() -> ("Value"=w215:T1)  [unwired: 2 in, 2 out]
              n175 = property on="Zn bubbler" class="Clust (strict)"() -> ("Value"=w209:T1)  [unwired: 2 in, 2 out]
              n176 = property on="Al bubbler" class="Clust (strict)"() -> ("Value"=w216:T2)  [unwired: 2 in, 2 out]
              n177 = property on="In bubbler" class="Clust (strict)"() -> ("Value"=w214:T2)  [unwired: 2 in, 2 out]
              n178 = property on="P gas" class="Clust (strict)"() -> ("Value"=w213:T2)  [unwired: 2 in, 2 out]
              n179 = property on="Se bubbler" class="Clust (strict)"() -> ("Value"=w210:T1)  [unwired: 2 in, 2 out]
              n180 = property on="As gas" class="Clust (strict)"() -> ("Value"=w212:T2)  [unwired: 2 in, 2 out]
              n181 = property on="P bubbler" class="Clust (strict)"() -> ("Value"=w211:T2)  [unwired: 2 in, 2 out]
              n182 = call "Set_V_III.vi"("Se bubbler"=w210, "P bubbler"=w211, "As gas"=w212, "P gas"=w213, "Run Started"=FALSE, "Zn bubbler"=w209, "In bubbler"=w214, "Ga bubbler"=w215, "Al bubbler"=w216) -> ()  [unwired: 3 in]
            }
          }
          n183 = property on="Argument List Out" class="Arr (strict)"("Value"=w200) -> ()  [unwired: 2 in, 2 out]
        }
        frame "Run" {
          n184 = property on="source array" class="Arr (strict)"() -> ("Value"=w218:refnum<vi>[])  [unwired: 2 in, 2 out]
          n185 = stacked-sequence {
            tunnel: w220 -> [_ w225 _ _]
            tunnel: w219 -> [_ _ _ w257]
            tunnel: w218 -> [_ _ w227 _]
            frame #0 {
              n186 = property on="Argument List Out" class="Arr (strict)"() -> ("Value"=w222:string[])  [unwired: 2 in, 2 out]
              n187 = call "Get_Argument.vi"("Argument"="run_started", "Argument List"=w222) -> ("Enabled"=w221:bool)
              n188 = property on="run started" class="Bool (strict)"("Value"=w221) -> ()  [unwired: 2 in, 2 out]
            }
            frame #1 {
              n189 = property on="prep_time" class="DigNum (strict)"() -> ("Value"=w226:dbl)  [unwired: 2 in, 2 out]
              n190 = Greater Or Equal?(x=w225, y=w226) -> (x >= y?=w224:bool)
              n191 = property on="prep_done" class="Bool (strict)"("Value"=w224) -> ()  [unwired: 2 in, 2 out]
            }
            frame #2 {
              n192 = property on="run started" class="Bool (strict)"() -> ("Value"=w228:bool)  [unwired: 2 in, 2 out]
              n193 = Not(x=w228) -> (.not. x?=w230:bool)
              n194 = for {
                shift-right: [w242] -> _
                shift-left: TRUE ("first") -> [w240]
                tunnel: w230 -> [w241]
                tunnel: w227 -> [w234] mode=indexing
                w233 = refnum<vi> refnum  # Cluster
                n195 = To More Specific Class(target class=w233, reference=w234) -> (specific class reference=w232:refnum<vi>)  [unwired: 1 in, 1 out]
                n196 = property class="Clust"(reference=w232) -> ("Controls[]"=w236:refnum<vi>[])  [unwired: 1 in, 2 out]
                n197 = Array Size(array=w236) -> (size(s)=w235:i32)
                n198 = case shown="6" w235 {
                  tunnel: [w249 w252] -> w238
                  tunnel: w232 -> [w249 w250]
                  frame Default {
                  }
                  frame 6 {
                    n199 = control-ref of="Ga bubbler"() -> (w251:refnum<vi>)
                    n200 = To More Specific Class(target class=w251, reference=w250) -> (specific class reference=w255:refnum<vi>)  [unwired: 1 in, 1 out]
                    n201 = property class="Clust (strict)"(reference=w255) -> ("Controls[]"=w254:refnum<vi>[])  [unwired: 1 in, 2 out]
                    n202 = Index Array(array=w254, index=5) -> (element=w252:refnum<vi>)
                  }
                }
                n203 = control-ref of="Al bubbler"() -> (w239:refnum<vi>)
                n204 = To More Specific Class(target class=w239, reference=w238) -> (specific class reference=w237:refnum<vi>)  [unwired: 1 in, 1 out]
                n205 = property class="Clust (strict)"(reference=w237) -> ("Value"=w248:T2)  [unwired: 1 in, 2 out]
                n206 = Unbundle By Name(w248) -> ("Prep"=w247:bool, "Run"=w246:bool, "Active"=w245:bool, "Name"=w231:string)
                n207 = property on="Status Out" class="Str"() -> ("Value"=w244:string)  [unwired: 2 in, 2 out]
                n208 = call "flow_strings.vi"("string in"=w244, "is first in?"=w240, "use source?"=w245, "name"=w231, "run source?"=w246, "prep source?"=w247, "is prep?"=w241) -> ("string out"=w243:string, "is first out?"=w242:bool)
                n209 = property on="Status Out" class="Str"("Value"=w243) -> ()  [unwired: 2 in, 2 out]
              }
            }
            frame #3 {
              n210 = property on="run started" class="Bool (strict)"() -> ("Value"=w259:bool)  [unwired: 2 in, 2 out]
              n211 = Not(x=w259) -> (.not. x?=w258:bool)
              n212 = property on="prep_done" class="Bool (strict)"() -> ("Value"=w260:bool)  [unwired: 2 in, 2 out]
              n213 = And(x=w260, y=w258) -> (x .and. y?=w256:bool)
              n214 = case shown="True" w256 {
                selector: w256 -> [_ w261]
                tunnel: w257 -> [_ w262]
                frame False {
                }
                frame True {
                  n215 = stacked-sequence {
                    tunnel: w262 -> [w264 _]
                    tunnel: w261 -> [w263 _]
                    frame #0 {
                      n216 = case shown="False" w264 {
                        tunnel: w263 -> [w273 _]
                        frame False {
                          n217 = property on="Ga bubbler" class="Clust (strict)"() -> ("Value"=w271:T1)  [unwired: 2 in, 2 out]
                          n218 = property on="In bubbler" class="Clust (strict)"() -> ("Value"=w270:T2)  [unwired: 2 in, 2 out]
                          n219 = property on="P gas" class="Clust (strict)"() -> ("Value"=w269:T2)  [unwired: 2 in, 2 out]
                          n220 = property on="Al bubbler" class="Clust (strict)"() -> ("Value"=w272:T2)  [unwired: 2 in, 2 out]
                          n221 = property on="Zn bubbler" class="Clust (strict)"() -> ("Value"=w265:T1)  [unwired: 2 in, 2 out]
                          n222 = property on="Se bubbler" class="Clust (strict)"() -> ("Value"=w266:T1)  [unwired: 2 in, 2 out]
                          n223 = property on="As gas" class="Clust (strict)"() -> ("Value"=w268:T2)  [unwired: 2 in, 2 out]
                          n224 = property on="P bubbler" class="Clust (strict)"() -> ("Value"=w267:T2)  [unwired: 2 in, 2 out]
                          n225 = call "Set_V_III.vi"("Se bubbler"=w266, "P bubbler"=w267, "As gas"=w268, "P gas"=w269, "Run Started"=w273, "Zn bubbler"=w265, "In bubbler"=w270, "Ga bubbler"=w271, "Al bubbler"=w272) -> ()  [unwired: 3 in]
                        }
                        frame True {
                        }
                      }
                    }
                    frame #1 {
                      n226 = property on="Argument List Out" class="Arr (strict)"() -> ("Value"=w274:string[])  [unwired: 2 in, 2 out]
                      n227 = call "Set_Argument.vi"("Enable"=TRUE, "Argument"="run_started", "Argument List In"=w274) -> ("Argument List Out"=w275:string[])
                      n228 = property on="Argument List Out" class="Arr (strict)"("Value"=w275) -> ()  [unwired: 2 in, 2 out]
                    }
                  }
                }
              }
            }
          }
        }
        frame "End" {
        }
        frame "Idle" {
        }
      }
    }
  }
